vi "Actor Core.vi"(8 "error in":errorcluster, 11 "Data Saver in":refnum<class "Data Saver.lvclass">) -> (0 "error out":errorcluster, 3 "Actor out":refnum<class "Actor.lvclass">)   [LabVIEW 2016, in "Data Saving.lvlib" / "Data Saver.lvclass"]
doc: "(<B>Filename</B>: Actor Framework.lvlib:Actor.lvclass:Actor Core.vi)\n\nReceives messages to the actor, reacts to them, and initiates any error handling that may shut the actor down.\n\nDescendant classes may override this VI to append parallel tasks for the actor to complete while it handles messages. Overrides use the Call Parent Method node."
uses:
  Data Saver.lvclass
  <vilib>/ActorFramework/Actor/Actor.lvclass
  <vilib>/express/express shared/transition.llb/Dynamic To Waveform Array.vi
  <vilib>/express/express signal manip/GetorSetDDTAttributes/Set DDT Attributes/SetT0.vi
  <vilib>/express/express shared/transition.llb/Waveform Array To Dynamic.vi
  <vilib>/express/express signal manip/GetorSetDDTAttributes/Set DDT Attributes/Set DDT Properties.xnode
  Abstract Saver/Abstract Saver.lvclass
panel:
  in  "Waveform Graph":dynamicdata(graph)
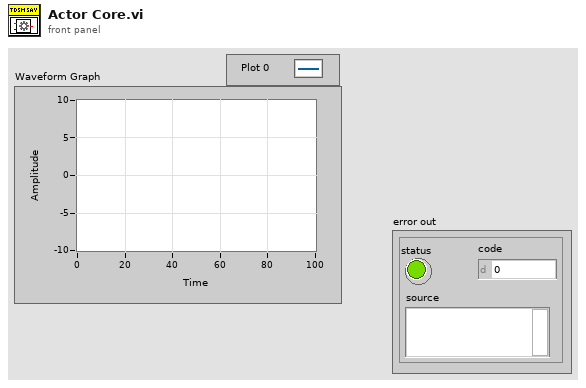
[diagram p1: front panel]
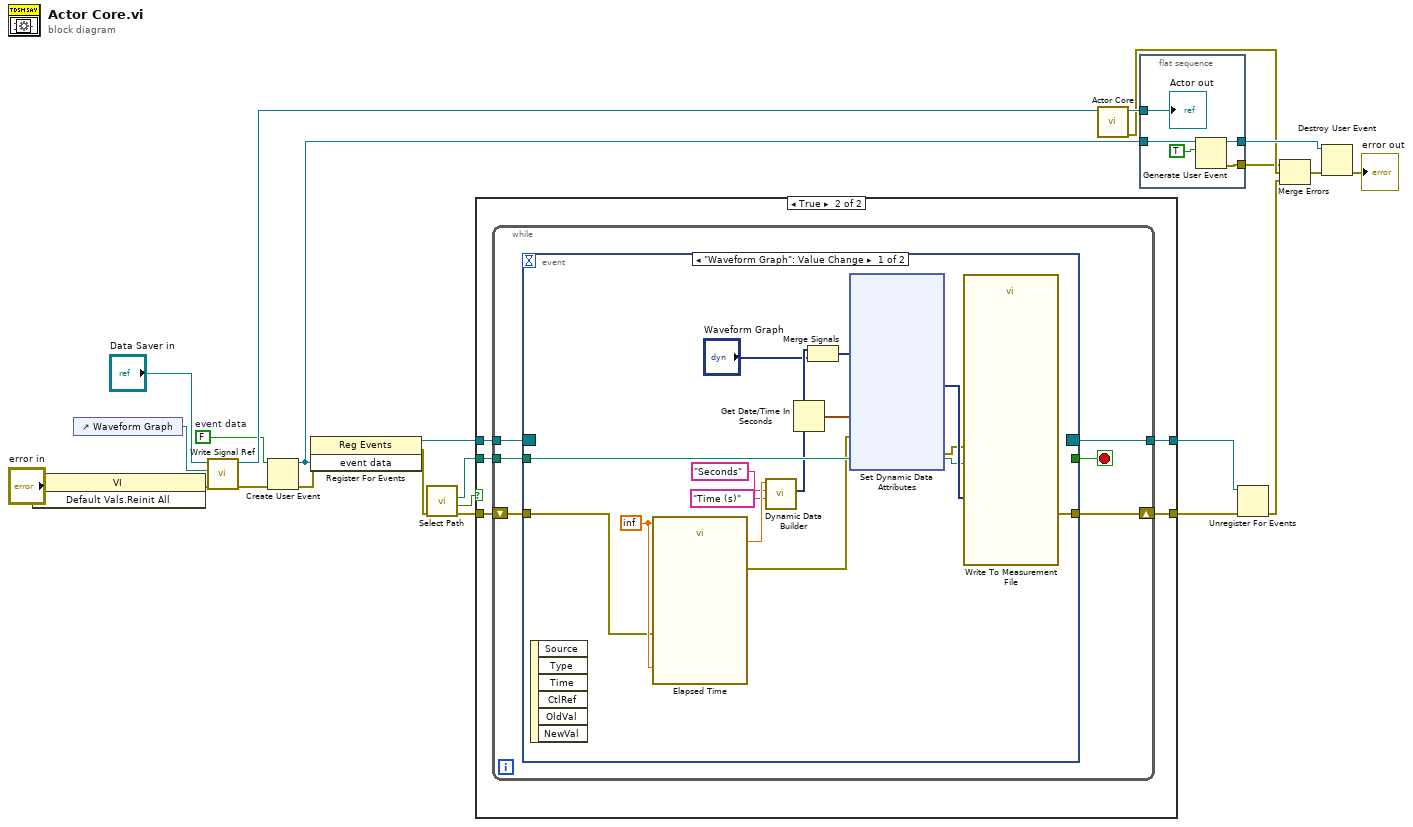
[diagram p0: block diagram]
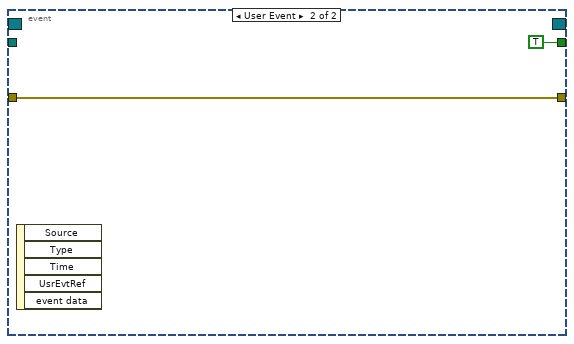
[diagram p3: hidden frame]
diagram:
  w16 = FALSE  # event data
  n1 = invoke class="VI" method="Default Vals.Reinit All"(error in="error in") -> (error out=w19:errorcluster)  [unwired: 2 in, 2 out]
  n2 = control-ref of="Waveform Graph"() -> (w18:refnum<vi>)
  n3 = call-dynamic "Write Signal Ref.vi"("error in (no error)"=w19, "Signal Ref"=w18, "Abstract Saver in"="Data Saver in") -> ("error out"=w15:errorcluster, "Abstract Saver out"=w21:refnum<class "Data Saver.lvclass">)  [unwired: 7 in]
  n4 = Create User Event(user event datatype=w16, error in=w15) -> (user event=w14:refnum<user-event>, error out=w17:errorcluster)
  n5 = register-events(error in=w17, w14) -> (reference out=w13:refnum<event-registration>, error out=w2:errorcluster)  [unwired: 1 in]
  n6 = call "Select Path.vi"("error in"=w2) -> ("error out"=w1:errorcluster, "Save?"=w3:bool, "selected path"=w4:path)  [unwired: 5 in, 1 out]
  n7 = case shown="True" w3 {
    tunnel: w13 -> [w25 w30]
    tunnel: [w25 w29] -> w10
    tunnel: w1 -> [w24 w28]
    tunnel: [w24 w27] -> w6
    tunnel: w4 -> [_ w26]
    frame False {
    }
    frame True {
      n8 = while {
        tunnel: w30 -> [w36]
        tunnel: [w35] -> w29
        shift-right: [w31] -> w27
        shift-left: w28 -> [w32]
        tunnel: w26 -> [w33]
        stop <- w34 stop-if-true
        n9 = event shown="[0] \"Waveform Graph\": Value Change" {
          selector: w36 -> [_ _]
          dyn-events: [_ _] -> w35
          timeout: _ -> [_ _]
          tunnel: [_ TRUE] -> w34
          tunnel: w33 -> [w46 _]
          tunnel: w32 -> [w42 w65]
          tunnel: [w37 w65] -> w31
          event "Waveform Graph": Value Change {
            w43 = inf
            n10 = event-data() -> ()  [unwired: 1 in, 6 out]
            n11 = call "Elapsed Time"("Time Target (s)"=w43, "error in (no error)"=w42, "Set Start Time (s)"=w43) -> ("Elapsed Time (s)"=w41:dbl, "error out"=w38:errorcluster)  [unwired: 9 in, 6 out]
            n12 = call "Dynamic Data Builder.vi"("Signal Name"="Time (s)", "Unit"="Seconds", "Number in"=w41) -> ("Dynamic Signame Out"=w45:dynamicdata)  [unwired: 8 in]
            n13 = Get Date/Time In Seconds() -> (seconds since 1Jan1904=w48:timestamp)
            n14 = Merge Signals(w45, "Waveform Graph") -> (w50:dynamicdata)
            n15 = xnode "Set Dynamic Data Attributes"("Signals In"=w50, "Timestamp"=w48, "error in"=w38) -> ("Signals Out"=w49:dynamicdata, "error out"=w47:errorcluster)  [unwired: 1 in]
            n16 = call "Write To Measurement File"("Signals"=w49, "error in (no error)"=w47, "Filename"=w46) -> ("error out"=w37:errorcluster)  [unwired: 14 in, 2 out]
          }
          event User Event {
            n17 = event-data() -> ()  [unwired: 1 in, 5 out]
          }
        }
      }
    }
  }
  n18 = call-parent "Actor Core.vi"("Actor in"=w21) -> ("error out"=w8:errorcluster, "Actor out"=w23:refnum<class "Actor.lvclass">)  [unwired: 9 in]
  n19 = flat-sequence {
    tunnel: w23 -> [w71]
    tunnel: w14 -> [w70]
    tunnel: [w68] -> w7
    tunnel: [w67] -> w9
    frame #0 {
      n20 = Generate User Event(user event=w70, event data cluster=TRUE ("event data")) -> (user event out=w67:refnum<user-event>, error out=w68:errorcluster)  [unwired: 2 in]
      "Actor out" <- w71
    }
  }
  n21 = Unregister For Events(event registration refnum=w10, error in=w6) -> (error out=w12:errorcluster)
  n22 = Merge Errors(w7, w8, w12) -> (w11:errorcluster)
  n23 = Destroy User Event(user event=w9, error in=w11) -> (error out=→"error out":errorcluster)
